vi "GVSGet Graph Ref to GraphNumber of DVIndex.vi"(10 "Graph Number":i32, 11 "DV Array index":i32) -> (1 "Frame VIRef":refnum<vi>, 2 "sQueueName":string, 3 "Inserted Graph VIRef out":refnum<vi>)   [LabVIEW 2013]
uses:
  GVSNew View Global.vi
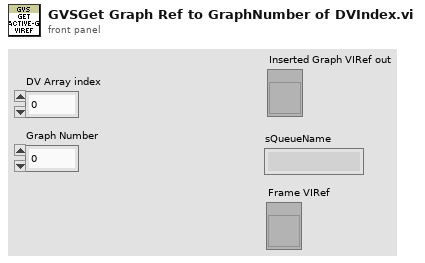
[diagram p1: front panel]
types:
  T1 = typedef "Graph Main Info Cluster.ctl" = cluster{"Selected_BarIdx":i32, "Selected_PanelIdx":i32, "Graph Main VIRef":refnum<vi>, "ToolBarClick":bool, "Spliter Ref Array":refnum<vi>[], "Panel Ref Array":refnum<vi>[], "Spliter_matrix":i32[][], "Panel_matrix":i32[][], "child_spliterIdx_matrix":i32[][], "split_pos_matrix":i32[][], "Title State":bool, "sQueueName":string, "Frame nID":i32, "Graph VIRef Array":cluster{"Graph VIRef":refnum<vi>, "Panel Idx":i32, "Frame VIRef":refnum<vi>, "Icon Ring":i32, "Graph Type":string}[], "View Type":string}
  T2 = cluster{"Graph VIRef":refnum<vi>, "Panel Idx":i32, "Frame VIRef":refnum<vi>, "Icon Ring":i32, "Graph Type":string}[]
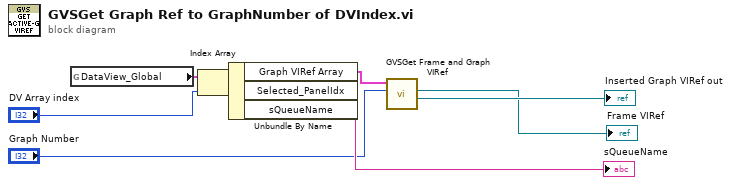
[diagram p0: block diagram]
diagram:
  n1 = global read "GVSNew View Global.vi" "DataView_Global"() -> (w8:T1[])
  n2 = Index Array(array=w8, index="DV Array index") -> (element=w7:T1)
  n3 = Unbundle By Name(w7) -> ("Graph VIRef Array"=w4:T2, "sQueueName"=→"sQueueName":string)  [unwired: 1 out]
  n4 = call "GVSGet Frame and Graph VIRef.vi"("Panel Idx"="Graph Number", "Graph VIRef Array"=w4) -> ("Graph VIRef"=→"Inserted Graph VIRef out":refnum<vi>, "Frame VIRef"=→"Frame VIRef":refnum<vi>)  [unwired: 5 in, 3 out]
